vi "Add.vi"(8 "error in (no error)":errorcluster, 10 "Runnable":refnum<class "Runnable.lvclass">, 11 "LUnit Test Suite In":refnum<class "LUnit Test Suite.lvclass">) -> (0 "error out":errorcluster, 3 "LUnit Test Suite Out":refnum<class "LUnit Test Suite.lvclass">)   [LabVIEW 2020, in "LUnit Test Suite.lvclass"]
uses:
  LUnit Test Suite.lvclass
  Core/Runnable/Runnable.lvclass
  LUnit Test Suite.lvclass/LUnit Test Suite.ctl
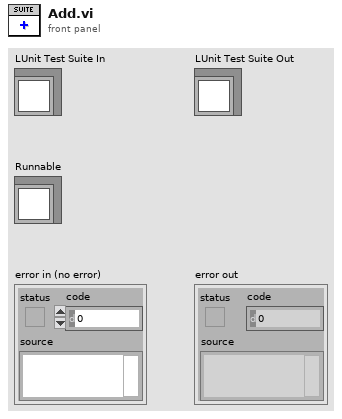
[diagram p1: front panel]
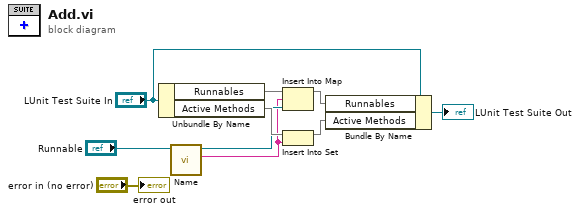
[diagram p0: block diagram]
diagram:
  n1 = Unbundle By Name("LUnit Test Suite In") -> ("Runnables"=w7:map{string, refnum<class "Runnable.lvclass">}, "Active Methods"=w3:set{string})
  n2 = call-dynamic "Name.vi"("Runnable in"="Runnable") -> ("Name"=w1:string, "Runnable out"=w2:refnum<class "Runnable.lvclass">)  [unwired: 8 in, 1 out]
  n3 = Insert Into Map(map in=w7, key=w1, value=w2) -> (map out=w6:map{string, refnum<class "Runnable.lvclass">})  [unwired: 2 out]
  n4 = Insert Into Set(10:w1, 11:w3) -> (3:w4:set{string})  [unwired: 1 out]
  n5 = Bundle By Name(cluster="LUnit Test Suite In", "Runnables"=w6, "Active Methods"=w4) -> (→"LUnit Test Suite Out":refnum<class "LUnit Test Suite.lvclass">)
  "error out" <- "error in (no error)"
